vi "Unflatten Value.vi"(8 "error in (no error)":errorcluster, 10 "Value":string, 11 "Boolean in":refnum<class "String 1D.lvclass">) -> (0 "error out":errorcluster, 3 "Boolean out":refnum<class "String 1D.lvclass">)   [LabVIEW 2017, in "String 1D.lvclass"]
uses:
  <vilib>/gpm_packages/@cs/data-type-serializer/source/String 1D/String 1D.lvclass
  <vilib>/gpm_packages/@cs/data-type-serializer/source/String 1D/String 1D.lvclass/String 1D.ctl
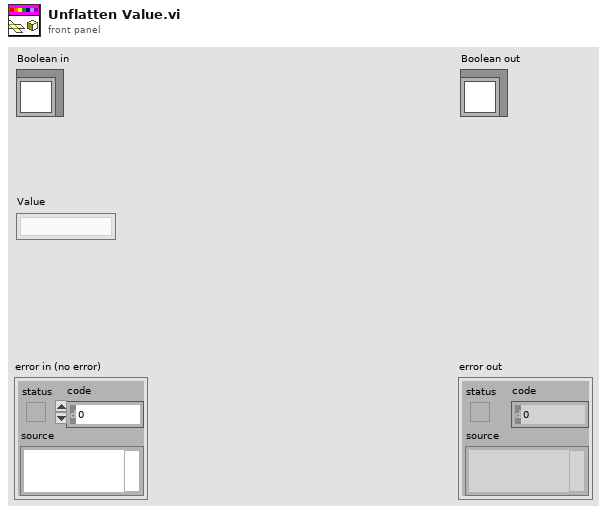
[diagram p1: front panel]
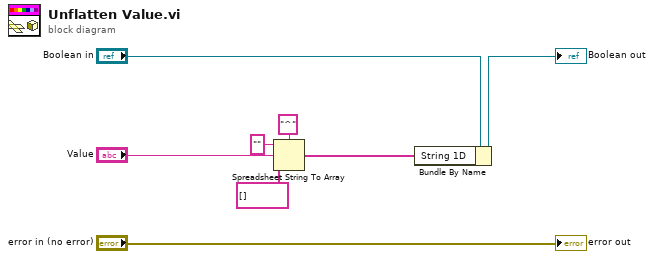
[diagram p0: block diagram]
diagram:
  n1 = Spreadsheet String To Array(delimiter (Tab)="^", format string="", spreadsheet string="Value", array type (2D Dbl)=string[] []) -> (array=w2:string[])
  n2 = Bundle By Name(cluster="Boolean in", "String 1D"=w2) -> (→"Boolean out":refnum<class "String 1D.lvclass">)
  "error out" <- "error in (no error)"
